vi "FdxTranslateErrorWordCvi.vi"(8 "error in":errorcluster, 11 "ErrorInfo":T1 {"ErrWord" items=["FDX_TRAFFIC_SHAP_ERROR"=0, "FDX_SEQUENCE_NO_ERROR"=0, "FDX_VL_FRAME_SIZE_ERRORFDX_VL_FRAME_SIZE_ERROR"=0, "FDX_SHORT_FRAME_ERROR"=0, "FDX_LONG_FRAME_ERROR"=0, "FDX_NO_VALID_SFD"=0, "FDX_MAC_ERROR"=0, "FDX_IP_ERROR"=0, "FDX_SHORG_IFG_ERROR"=0, "FDX_CRC_ERROR"=0, "FDX_TRIP_NIBBLE_ERROR"=0, "FDX_PREAMBLE_ERROR"=0, "FDX_RX_ERROR"=0]}) -> (0 "error out":errorcluster, 3 "ErrStr":string)   [LabVIEW 2020, in "AIM664LV.lvlib"]
doc: "This function translates a Firmware specific Error Report Word into a string, containing 3-character wide abbreviations for the corresponding errors."
uses:
  AIM664LV.lvlib
  AFDX_LibraryAdmin/FdxGlobalDllPath.vi
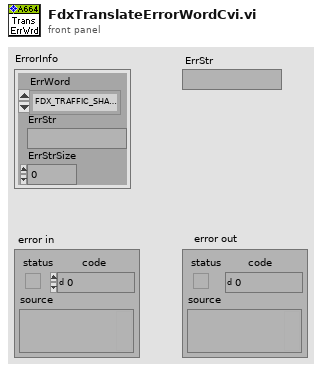
[diagram p1: front panel]
types:
  T1 = cluster{"ErrWord":u16, "ErrStr":string, "ErrStrSize":u8}
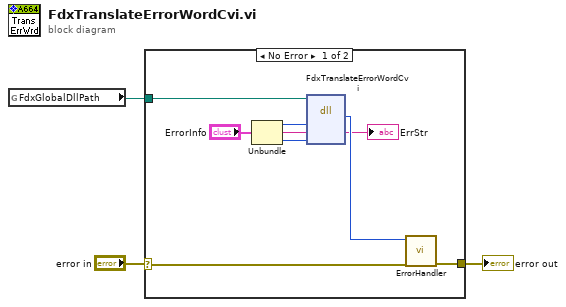
[diagram p0: block diagram]
diagram:
  n1 = global read "FdxGlobalDllPath.vi" "FdxGlobalDllPath"() -> (w1:path)
  n2 = case shown="No Error" "error in" {
    selector: "error in" -> [w11 w13]
    tunnel: [w12 w13] -> w3
    tunnel: w1 -> [w4 _]
    frame No Error {
      n3 = Unbundle("ErrorInfo") -> ("ErrWord"=w7:u16, "ErrStr"=w6:string, "ErrStrSize"=w5:u8)
      n4 = dll-call lib="aim_fdx.19.dll" fn="FdxTranslateErrorWordCvi"(path in=w4, "ErrWord"=w7, "ErrStr"=w6, "ErrStrSize"=w5) -> ("status"=w10:i32, "ErrStr"=→"ErrStr":string)  [unwired: 4 in, 2 out]
      n5 = call "ErrorHandler.vi"("error in"=w11, "AIM Error"=w10) -> ("error out"=w12:errorcluster)  [unwired: 9 in]
    }
    frame Error {
    }
  }
  "error out" <- w3
